vi "Read Parameter R Table.vi"(8 "error in (no error)":errorcluster, 11 "1553 SubComponent in":refnum<class "1553 SubComponent.lvclass">) -> (0 "error out":errorcluster, 2 "Parameter R Table":refnum<class "Registry.lvclass">, 3 "1553 SubComponent out":refnum<class "1553 SubComponent.lvclass">)   [LabVIEW 2020, in "BCI-1553 API.lvlib" / "1553 SubComponent.lvclass"]
uses:
  1553 SubComponent.lvclass
  Dependencies/Registry/Registry.lvclass
  1553 SubComponent.lvclass/1553 SubComponent.ctl
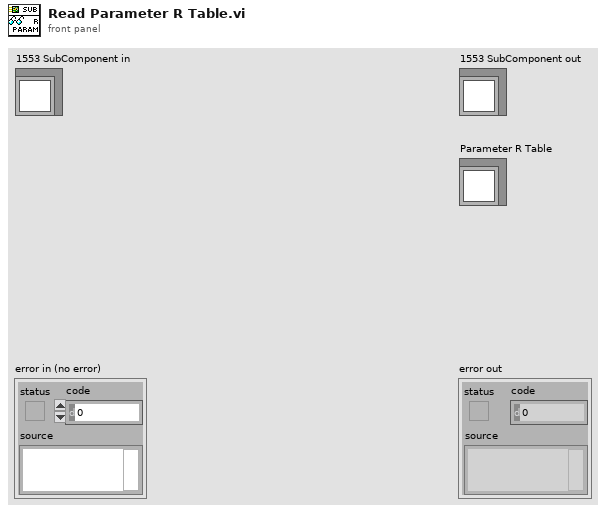
[diagram p1: front panel]
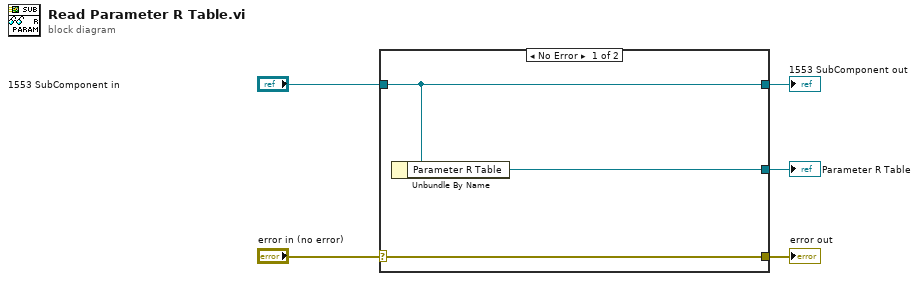
[diagram p0: block diagram]
diagram:
  n1 = case shown="No Error" "error in (no error)" {
    selector: "error in (no error)" -> [w8 w9]
    tunnel: [w8 w9] -> w4
    tunnel: [w7 w10] -> w2
    tunnel: "1553 SubComponent in" -> [w7 w10]
    tunnel: [w6 _] -> w1
    frame No Error {
      n2 = Unbundle By Name(w7) -> ("Parameter R Table"=w6:refnum<class "Registry.lvclass">)
    }
    frame Error {
    }
  }
  "error out" <- w4
  "1553 SubComponent out" <- w2
  "Parameter R Table" <- w1
